vi "Create Circle on Image Center.vi"(1 "X Resolution":i32, 2 "Y Resolution":i32) -> (0 "circle center":cluster{dbl, dbl})   [LabVIEW 2010]
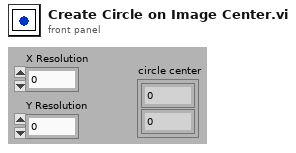
[diagram p1: front panel]
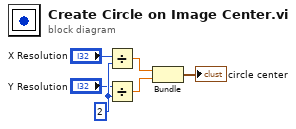
[diagram p0: block diagram]
diagram:
  w6 = 2 ("y")
  n1 = Divide(x="X Resolution", y=w6) -> (x/y=w3:dbl)
  n2 = Divide(x="Y Resolution", y=w6) -> (x/y=w2:dbl)
  n3 = Bundle(w3, w2) -> (→"circle center":cluster{dbl, dbl})  [unwired: 1 in]
